vi "Init XNET Cyclic_Status Session.vi"(8 "error in (no error)":errorcluster, 11 "DUT Sample in":refnum<class "DUT Sample.lvclass">) -> (0 "error out":errorcluster, 3 "DUT Sample out":refnum<class "DUT Sample.lvclass">)   [LabVIEW 2023, in "DUT Sample.lvclass"]
uses:
  DUT Sample.lvclass
  DUT Sample.lvclass/DUT Sample.ctl
  <vilib>/xnet/xnet.llb/XNET Create Session (Signal Output Single-point).vi
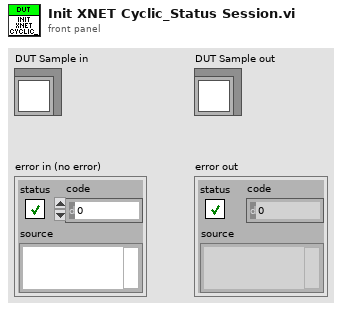
[diagram p1: front panel]
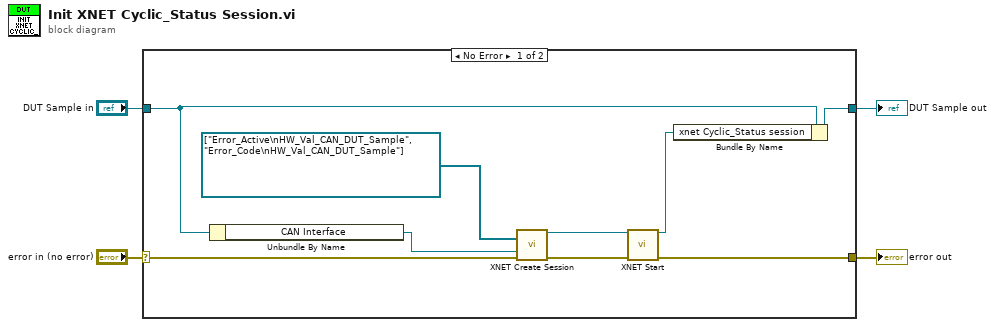
[diagram p0: block diagram]
diagram:
  n1 = case shown="No Error" "error in (no error)" {
    selector: "error in (no error)" -> [w10 w15]
    tunnel: [w9 w15] -> w3
    tunnel: [w8 w14] -> w1
    tunnel: "DUT Sample in" -> [w6 w14]
    frame No Error {
      n2 = Unbundle By Name(w6) -> ("CAN Interface"=w5:refnum<k21>)
      n3 = call-poly <vilib>:"XNET Create Session.vi"("signal list"=refnum<k21>[] ["Error_Active\nHW_Val_CAN_DUT_Sample", "Error_Code\nHW_Val_CAN_DUT_Sample"] ("Select Signal List from database"), "interface"=w5, "error in (no error)"=w10) -> ("session out"=w12:refnum<k21>, "error out"=w11:errorcluster)  [unwired: 11 out]
      n4 = call <vilib>:"XNET Start.vi"("session in"=w12, "error in (no error)"=w11) -> ("session out"=w7:refnum<k21>, "error out"=w9:errorcluster)  [unwired: 12 in]
      n5 = Bundle By Name(cluster=w6, "xnet Cyclic_Status session"=w7) -> (w8:refnum<class "DUT Sample.lvclass">)
    }
    frame Error {
    }
  }
  "error out" <- w3
  "DUT Sample out" <- w1
